vi "OPC UA Server with Historical Data.vi"() -> ()   [LabVIEW 2017]
uses:
  <vilib>/OPCUA/controls/Historical Access.ctl
  <vilib>/OPCUA/NI OPC UA Server.lvlib
panel:
  out "Item Node Id":string="ns=2;s=Process Data.Temperature"
  in  "Stop Button":bool
  out "Server Endpoint URL":string="opc.tcp://XPS15HPH:49580"
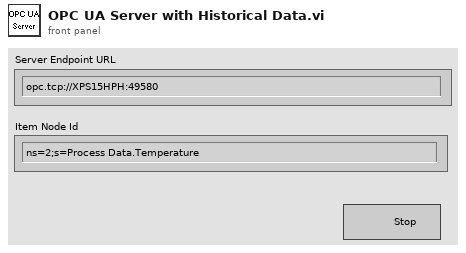
[diagram p1: front panel]
types:
  T1 = typedef "Historical Access.ctl" = cluster{"enable":bool, "queue size (1000)":u32}
  T2 = cluster{"name":string, "data type":u16, "access level":u16, "description":string}
  T3 = typedef "OPC UA Server Refnum.ctl" = refnum<k21>
  T4 = typedef "NodeId.ctl" = string
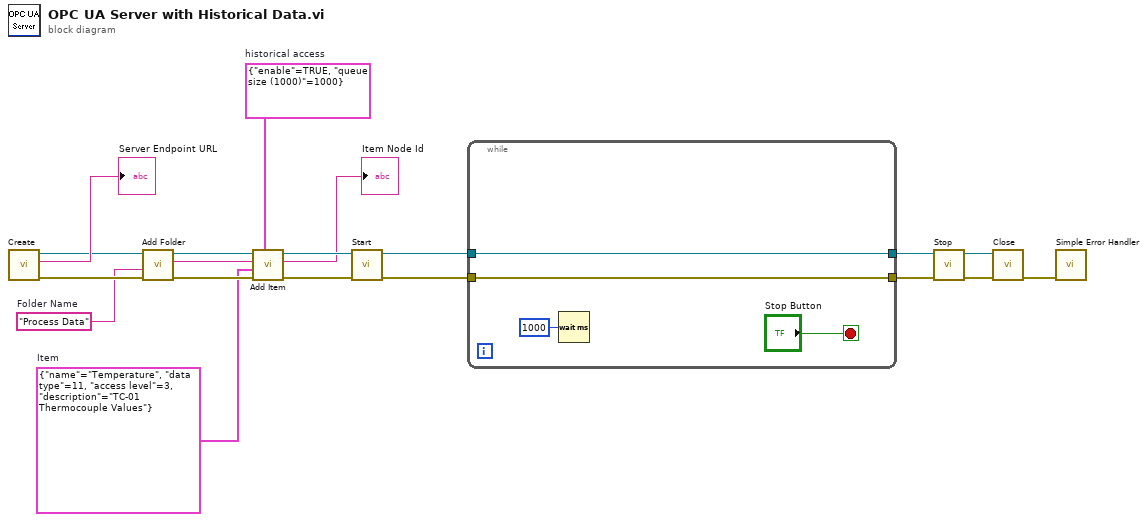
[diagram p0: block diagram]
diagram:
  w1 = T1 {"enable"=TRUE, "queue size (1000)"=1000}  # historical access
  w6 = T2 {"name"="Temperature", "data type"=11, "access level"=3, "description"="TC-01 Thermocouple Values"}  # Item
  w13 = "Process Data"  # Folder Name
  n1 = call <vilib>:"Create.vi"() -> ("error out"=w19:errorcluster, "server endpoint URL"=→"Server Endpoint URL":string, "OPC UA server refnum out"=w12:T3)  [unwired: 9 in]
  n2 = call <vilib>:"Add Folder.vi"("error in (no error)"=w19, "folder name"=w13, "OPC UA server refnum in"=w12) -> ("error out"=w18:errorcluster, "folder node ID"=w7:T4, "OPC UA server refnum out"=w11:T3)  [unwired: 5 in]
  n3 = call <vilib>:"Add Item.vi"("historical access"=w1, "error in (no error)"=w18, "item"=w6, "parent folder node ID"=w7, "OPC UA server refnum in"=w11) -> ("error out"=w8:errorcluster, "item node ID"=→"Item Node Id":T4, "OPC UA server refnum out"=w9:T3)  [unwired: 2 in, 1 out]
  n4 = call <vilib>:"Start.vi"("error in (no error)"=w8, "OPC UA server refnum in"=w9) -> ("error out"=w17:errorcluster, "OPC UA server refnum out"=w10:T3)  [unwired: 7 in, 1 out]
  n5 = while {
    tunnel: w17 -> [w20]
    tunnel: w10 -> [w21]
    tunnel: [w21] -> w3
    tunnel: [w20] -> w2
    stop <- "Stop Button" stop-if-true
    n6 = Wait (ms)(milliseconds to wait=u32 1000) -> ()  [unwired: 1 out]
  }
  n7 = call <vilib>:"Stop.vi"("error in (no error)"=w2, "OPC UA server refnum in"=w3) -> ("error out"=w15:errorcluster, "OPC UA server refnum out"=w5:T3)  [unwired: 8 in]
  n8 = call <vilib>:"Close.vi"("error in (no error)"=w15, "OPC UA server refnum in"=w5) -> ("error out"=w14:errorcluster)  [unwired: 9 in]
  n9 = call <vilib>:"Simple Error Handler.vi"("error in (no error)"=w14) -> ()  [unwired: 4 in, 5 out]
